vi "Delete Timings Header.vi"(8 "error in (no error)":errorcluster, 11 "Save Image in":refnum<class "Save Image.lvclass">) -> (0 "error out":errorcluster, 3 "Save Image out":refnum<class "Save Image.lvclass">)   [LabVIEW 2018, in "Save Image.lvclass"]
uses:
  Save Image.lvclass
  Save Image.lvclass/Save Image.ctl
  Simulated_Header/Simulated_Header.lvclass
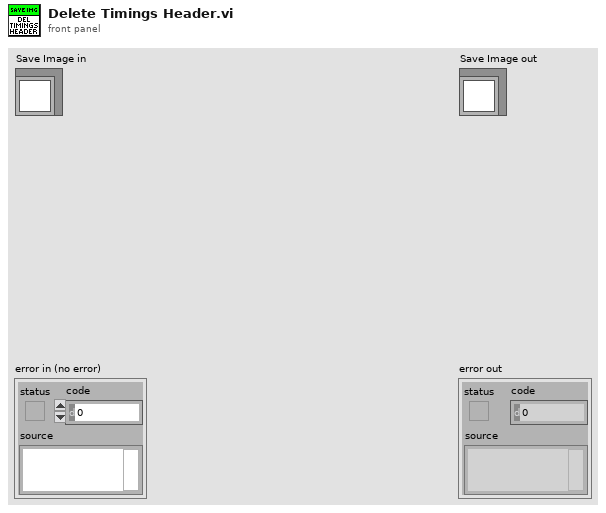
[diagram p1: front panel]
types:
  T1 = cluster{"Image Path":string, "Image Name":string, "Image Delays":string[]}
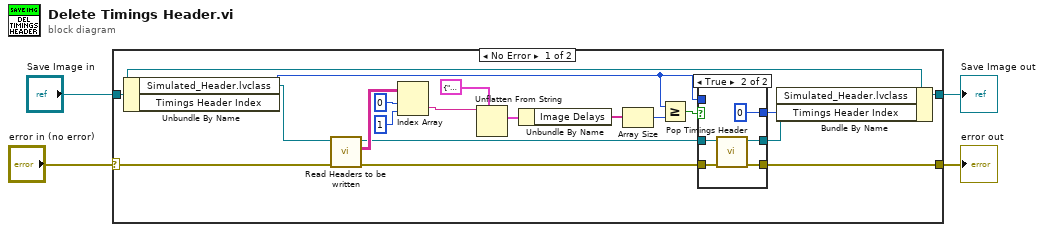
[diagram p0: block diagram]
diagram:
  n1 = case shown="No Error" "error in (no error)" {
    selector: "error in (no error)" -> [w17 w33]
    tunnel: [w20 w33] -> w2
    tunnel: [w22 w32] -> w1
    tunnel: "Save Image in" -> [w23 w32]
    frame No Error {
      n2 = Unbundle By Name(w23) -> ("Simulated_Header.lvclass"=w18:refnum<class "Simulated_Header.lvclass">, "Timings Header Index"=w5:u16)
      n3 = call "Read Headers to be written.vi"("error in (no error)"=w17, "Header in"=w18) -> ("error out"=w6:errorcluster, "Headers to be written"=w16:string[][], "Header out"=w7:refnum<class "Simulated_Header.lvclass">)  [unwired: 7 in]
      n4 = Index Array(array=w16, index (row)=0, index (col)=1) -> (element=w13:string)
      n5 = Unflatten From String(type=T1 {"Image Path"="", "Image Name"="", "Image Delays"=[]} ("Image Delays Settings"), binary string=w13) -> (value=w11:T1)  [unwired: 3 in, 2 out]
      n6 = Unbundle By Name(w11) -> ("Image Delays"=w10:string[])
      n7 = Array Size(array=w10) -> (size(s)=w9:i32)
      n8 = Greater Or Equal?(x=w5, y=w9) -> (x >= y?=w8:bool)
      n9 = case shown="True" w8 {
        tunnel: [w25 w31] -> w21
        tunnel: [w26 w30] -> w20
        tunnel: [w24 u8 0] -> w19
        tunnel: w7 -> [w25 w28]
        tunnel: w6 -> [w26 w27]
        tunnel: w5 -> [w24 _]
        frame False {
        }
        frame True {
          n10 = call "Pop Timings Header.vi"("error in (no error)"=w27, "Header in"=w28) -> ("error out"=w30:errorcluster, "Header out"=w31:refnum<class "Simulated_Header.lvclass">)  [unwired: 7 in, 1 out]
        }
      }
      n11 = Bundle By Name(cluster=w23, "Simulated_Header.lvclass"=w21, "Timings Header Index"=w19) -> (w22:refnum<class "Save Image.lvclass">)
    }
    frame Error {
    }
  }
  "error out" <- w2
  "Save Image out" <- w1
